vi "Memory.Array.Get Number of Elements.vi"(8 "error in (no error)":errorcluster, 11 "Memory.Array in":refnum<class "Memory.Array.lvclass">) -> (0 "error out":errorcluster, 2 "number of elements":u64, 3 "Memory.Array out":refnum<class "Memory.Array.lvclass">)   [LabVIEW 2016, in "LabVIEW Memory Manager.lvlib" / "Memory.Array.lvclass"]
uses:
  Memory.Array.lvclass
  Memory.Array.lvclass/Memory.Array.ctl
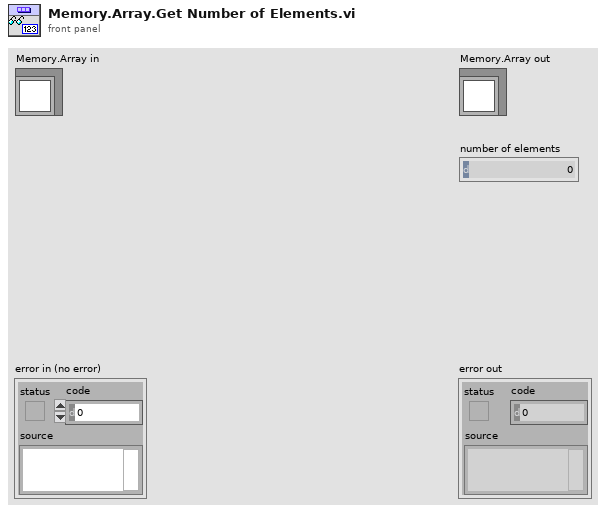
[diagram p1: front panel]
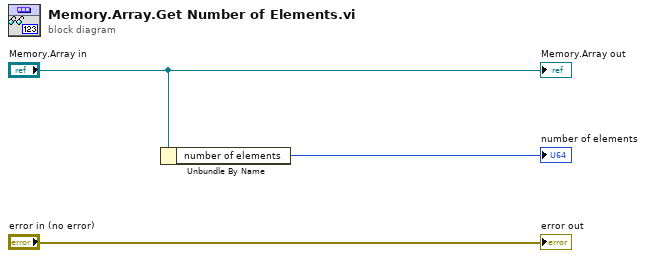
[diagram p0: block diagram]
diagram:
  n1 = Unbundle By Name("Memory.Array in") -> ("number of elements"=→"number of elements":u64)
  "error out" <- "error in (no error)"
  "Memory.Array out" <- "Memory.Array in"
